vi "NItest.vi"(5 "Coupling":u16(ring)=2 items=["DC 1 MOhm", "AC 1 MOhm", "DC 50 Ohm", "AC 50 OHM"], 6 "RF data Sampling":T2={"Sampling Rate"=0, "Delay (micro s)"=0.0, "rf points per line"=500} {"Delay (micro s)" format="%.2f"}, 7 "Boolean":bool=TRUE) -> (0 "voltage range":T1, 1 "Equivalent delay\ndistance (mm)":dbl=1.5 format="%.2f", 2 "RF data Out":T2 {"Delay (micro s)" format="%.2f"}, 3 "ID":refnum<k15>)   [LabVIEW 2022 SP3]
uses:
  Instance          14 12Saved   test .vi
  <instrlib>/niScope/Acquire/Fetch/niScope Fetch.vi
  Instance          15 12Saved   test .vi
panel:
  out "Nominal Samples":i32
  out "Samping Rate":dbl format="%.2f"
  in  "ExitSendCmd":bool
  in  "Voltage Scale":u16(ring)
  in  "Time scale per Div":i32(ring)=8 items=["100 ns", "200 ns", "500 ns", "1 micros", "2 micros", "5 micros", "10 micros", "20 micros", "50 micros", "100 micros", "200 micros", "500 micros", "1 ms", "2 ms", "5 ms", "10 ms", "20 ms", "50 ms", "100 ms", "200 ms"]
  out "Waveform Graph":cluster{i32, dbl, "wfm":dbl[]}(graph)
  out "errorMessage":string
  in  "Trigger":T3={"Source"=1, "Coupling"=0, "Slope"=0, "Level (% CH1 or mV Ext)"=1000.0} {"Slope" items=["Positive", "Negative"]; "Level (% CH1 or mV Ext)" format="%.2f"; "Coupling" items=["DC 1 MOhm", "AC 1 MOhm", "DC 50 Ohm", "AC 50 Ohm"]; "Source" items=["Chan 1", "External"]}
  # "Take out option of changing offset.  Move in time scale selector."
  # "Red line indicates last pt of RF data"
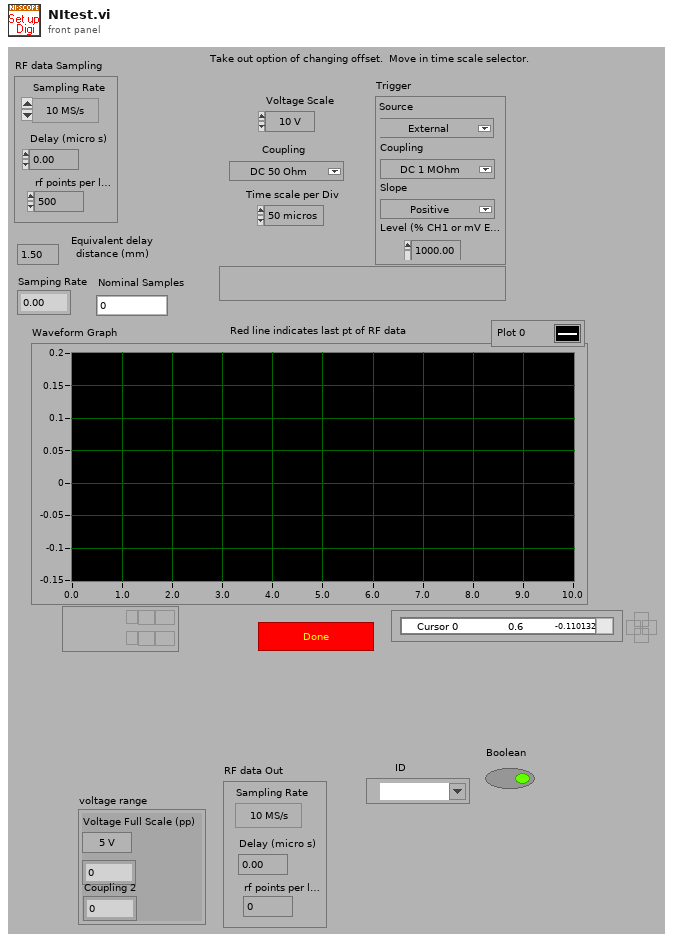
[diagram p1: front panel]
types:
  T1 = cluster{"Voltage Full Scale (pp)":u16, i32, "Coupling 2":u16}
  T2 = cluster{"Sampling Rate":u16, "Delay (micro s)":dbl, "rf points per line":u16}
  T3 = cluster{"Source":u16, "Coupling":u16, "Slope":u16, "Level (% CH1 or mV Ext)":dbl}
  T4 = cluster{"Voltage Scale":u16, i32, "Coupling":u16}
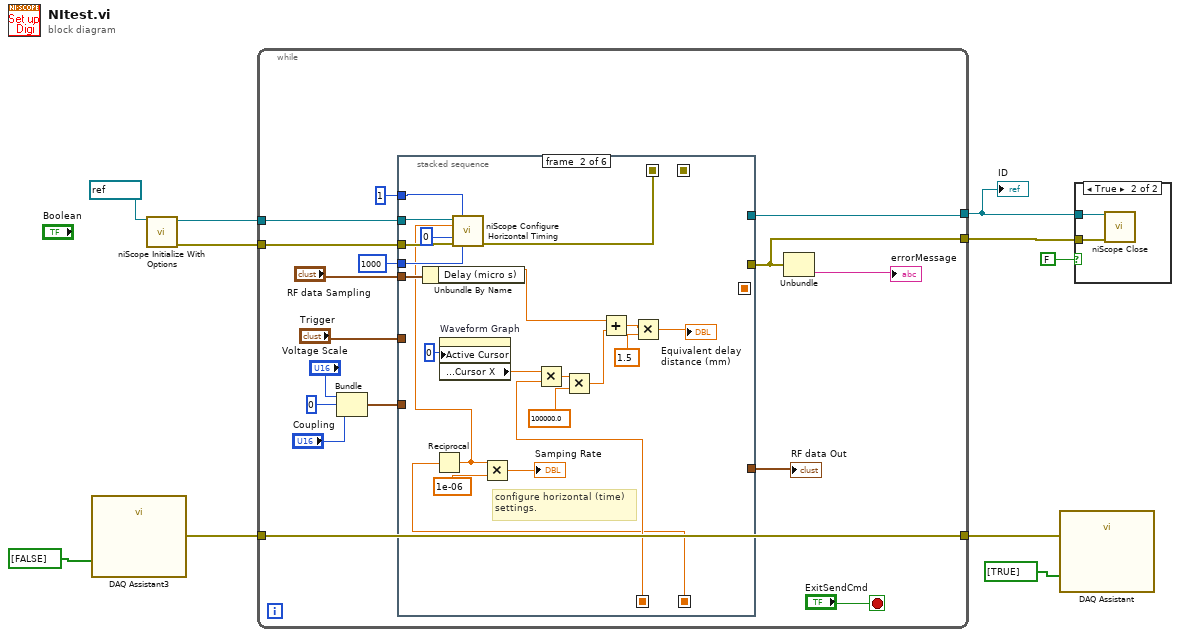
[diagram p0: block diagram]
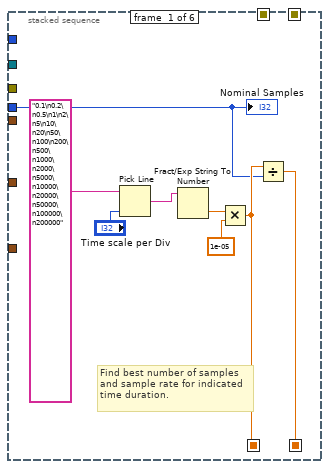
[diagram p3: hidden frame]
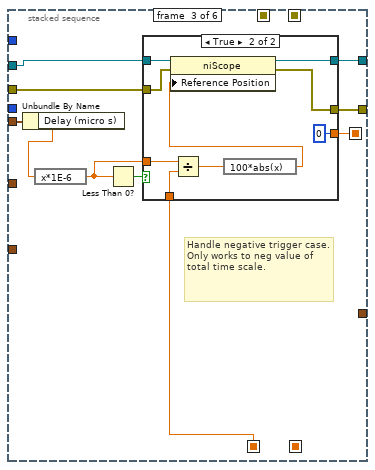
[diagram p4: hidden frame]
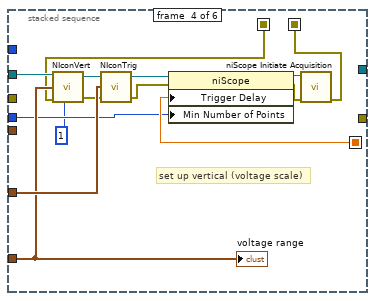
[diagram p6: hidden frame]
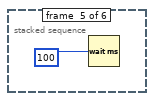
[diagram p7: hidden frame]
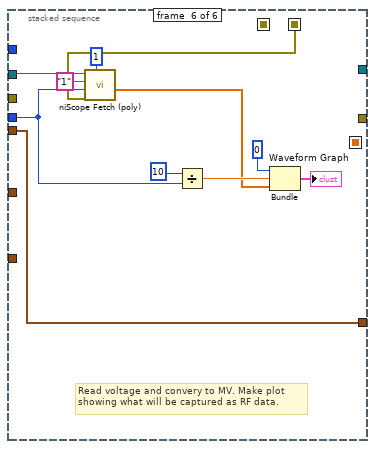
[diagram p8: hidden frame]
diagram:
  n1 = call "DAQ Assistant3"("data"=bool[] [FALSE]) -> ("error out"=w7:errorcluster)  [unwired: 3 in, 15 out]
  n2 = call <instrlib>:"niScope Initialize With Options.vi"("resource name"=refnum<k15> "Dig1") -> ("instrument handle"=w9:refnum<k15>, "error out"=w10:errorcluster)  [unwired: 4 in, 9 out]
  n3 = while {
    tunnel: w10 -> [w24]
    tunnel: w9 -> [w23]
    tunnel: [w14] -> w6
    tunnel: w7 -> [w14]
    tunnel: [w11] -> w2
    tunnel: [w12] -> w4
    stop <- "ExitSendCmd" stop-if-true
    n4 = Bundle("Voltage Scale"="Voltage Scale", 0, "Coupling"="Coupling") -> (w16:T4)  [unwired: 1 out]
    n5 = stacked-sequence {
      seq-local: [w28 _ _ _ _ _] -> [_ w42 _ _ _ _]
      seq-local: [_ _ _ w85 _ _] -> [_ _ _ _ _ w97]
      seq-local: [_ w35 _ _ _ _] -> [_ _ _ w86 _ _]
      seq-local: [w29 _ _ _ _ _] -> [_ w45 w58 _ _ _]
      seq-local: [_ _ w64 _ _ _] -> [_ _ _ w80 _ _]
      tunnel: w23 -> [_ w41 w63 w87 _ w96]
      tunnel: "RF data Sampling" -> [_ w54 w65 _ _ w95]
      tunnel: [_ _ _ _ _ w95] -> w26
      tunnel: "Trigger" -> [_ _ _ w91 _ _]
      tunnel: 1 -> [_ w39 _ _ _ _]
      tunnel: 1000 -> [w27 w40 _ w79 _ w94]
      tunnel: w24 -> [_ w38 w62 _ _ _]
      tunnel: w16 -> [_ _ _ w88 _ _]
      tunnel: [_ _ w60 _ _ _] -> w12
      tunnel: [_ _ w61 _ _ _] -> w11
      frame #0 {
        # "Find best number of samples\nand sample rate for indicated\ntime duration."
        n6 = Pick Line(multi-line string="0.1\n0.2\n0.5\n1\n2\n5\n10\n20\n50\n100\n200\n500\n1000\n2000\n5000\n10000\n20000\n50000\n100000\n200000" ("ResourceName"), line index="Time scale per Div") -> (output string=w34:string)  [unwired: 1 out]
        n7 = Fract/Exp String To Number(string=w34) -> (number=w32:dbl)  [unwired: 1 in, 3 out]
        n8 = Multiply(x=w32, y=1e-05) -> (x*y=w29:dbl)
        n9 = Divide(x=w29, y=w27) -> (x/y=w28:dbl)
        "Nominal Samples" <- w27
      }
      frame #1 {
        # "configure horizontal (time)\nsettings."
        n10 = Unbundle By Name(w54) -> ("Delay (micro s)"=w50:dbl)
        n11 = Reciprocal(x=w42) -> (1/x=w36:dbl)
        n12 = property on="Waveform Graph" class="WFGraph (strict)"("Active Cursor"=0) -> ("Cursor.Cursor Position:Cursor X"=w47:dbl)  [unwired: 2 in, 2 out]
        n13 = call <instrlib>:"niScope Configure Horizontal Timing.vi"("instrument handle"=w41, "number of records"=w39, "min sample rate"=w36, "reference position"=0, "error in"=w38, "min record length"=w40) -> ("error out"=w35:errorcluster)  [unwired: 1 in, 8 out]
        n14 = Multiply(x=w36, y=1e-06) -> (x*y=→"Samping Rate":dbl)
        n15 = Multiply(x=w47, y=w45) -> (x*y=w52:dbl)
        n16 = Multiply(x=w52, y=100000.0) -> (x*y=w46:dbl)
        n17 = Add(x=w50, y=w46) -> (x+y=w49:dbl)
        n18 = Multiply(x=w49, y=1.5) -> (x*y=→"Equivalent delay\ndistance (mm)":dbl)
      }
      frame #2 {
        # "Handle negative trigger case. Only works to neg value of total time scale."
        n19 = Unbundle By Name(w65) -> ("Delay (micro s)"=w57:dbl)
        n20 = expression code="x*1E-6"(w57) -> (w56:dbl)
        n21 = Less Than 0?(x=w56) -> (x < 0?=w59:bool)
        n22 = case shown="True" w59 {
          tunnel: [w66 0] -> w64
          tunnel: w63 -> [w68 w77]
          tunnel: w62 -> [w67 w76]
          tunnel: [w68 w75] -> w61
          tunnel: [w67 w74] -> w60
          tunnel: w58 -> [_ w73]
          tunnel: w56 -> [w66 w72]
          frame False {
          }
          frame True {
            n23 = Divide(x=w72, y=w73) -> (x/y=w70:dbl)
            n24 = expression code="100*abs(x)"(w70) -> (w69:dbl)
            n25 = property class="niScope"(reference=w77, error in=w76, "Reference Position"=w69) -> (reference out=w75:refnum<k15>, error out=w74:errorcluster)
          }
        }
      }
      frame #3 {
        # "set up vertical (voltage scale)"
        n26 = call "NIconVert.vi"("InstrumentID"=w87, "V scale"=w88, "error in"=w86, "Channel (0)"=1) -> ("Status"=w90:refnum<k15>, "error out"=w89:errorcluster)  [unwired: 2 out]
        n27 = call "NIconTrig.vi"("error in"=w89, "Trigger"=w91, "InstrumentID"=w90) -> ("error out"=w81:errorcluster, "dup id"=w84:refnum<k15>)  [unwired: 1 out]
        n28 = property class="niScope"(reference=w84, error in=w81, "Trigger Delay"=w80, "Min Number of Points"=w79) -> (reference out=w83:refnum<k15>, error out=w82:errorcluster)
        n29 = call <instrlib>:"niScope Initiate Acquisition.vi"("instrument handle"=w83, "error in"=w82) -> ("error out"=w85:errorcluster)  [unwired: 13 out]
        "voltage range" <- w88
      }
      frame #4 {
        n30 = Wait (ms)(milliseconds to wait=100) -> ()  [unwired: 1 out]
      }
      frame #5 {
        # "Read voltage and convery to MV. Make plot\nshowing what will be captured as RF data."
        n31 = call-poly <instrlib>:"niScope Fetch (poly).vi"("timeout"=1, "error in"=w97, "numSamples"=w94, "channels"="1", "instrument handle"=w96) -> ("wfm"=w99:dbl[])  [unwired: 6 out]
        n32 = Divide(x=10, y=w94) -> (x/y=w100:dbl)
        n33 = Bundle(0, w100, "wfm"=w99) -> (→"Waveform Graph":cluster{i32, dbl, "wfm":dbl[]})  [unwired: 1 out]
      }
    }
    "RF data Out" <- w26
    n34 = Unbundle(w12) -> ("source"=→"errorMessage":string)  [unwired: 2 out]
  }
  "ID" <- w2
  n35 = call "DAQ Assistant"("data"=bool[] [TRUE], "error in"=w6) -> ()  [unwired: 2 in, 16 out]
  n36 = case shown="True" FALSE {
    tunnel: w4 -> [_ w105]
    tunnel: w2 -> [_ w104]
    frame False {
    }
    frame True {
      n37 = call <instrlib>:"niScope Close.vi"("instrument handle"=w104, "error in"=w105) -> ()  [unwired: 14 out]
    }
  }
